vi "Stage_enable.vi"(8 "error in (no error)":errorcluster, 9 "Boolean":bool, 10 "Axes Select":u16(ring) items=["X", "Y", "Z"], 11 "reference":refnum<k7>) -> (0 "error out":errorcluster, 3 "reference out":refnum<k7>)   [LabVIEW 2020]
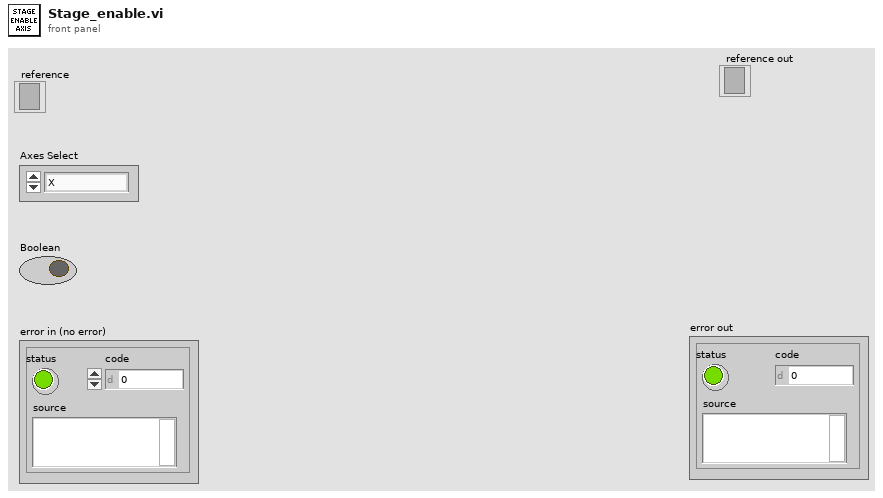
[diagram p1: front panel]
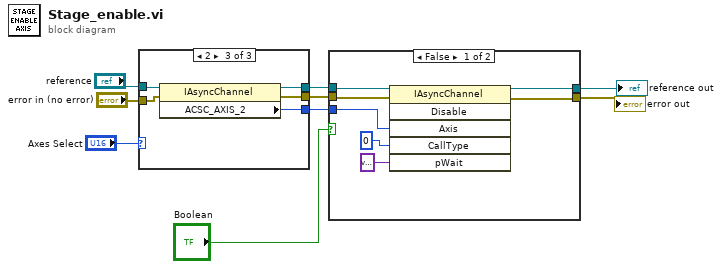
[diagram p0: block diagram]
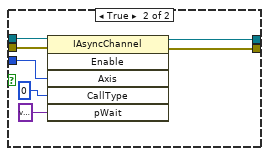
[diagram p2: hidden frame]
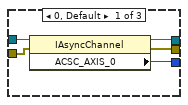
[diagram p3: hidden frame]
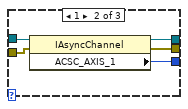
[diagram p4: hidden frame]
diagram:
  n1 = case shown="2" "Axes Select" {
    tunnel: [w14 w19 w24] -> w6
    tunnel: [w13 w18 w23] -> w5
    tunnel: [w12 w17 w22] -> w4
    tunnel: "reference" -> [w11 w16 w21]
    tunnel: "error in (no error)" -> [w10 w15 w20]
    frame 0, Default {
      n2 = property class="IAsyncChannel"(reference=w11, error in=w10) -> (reference out=w14:refnum<k7>, error out=w13:errorcluster, "ACSC_AXIS_0"=w12:i32)
    }
    frame 1 {
      n3 = property class="IAsyncChannel"(reference=w16, error in=w15) -> (reference out=w19:refnum<k7>, error out=w18:errorcluster, "ACSC_AXIS_1"=w17:i32)
    }
    frame 2 {
      n4 = property class="IAsyncChannel"(reference=w21, error in=w20) -> (reference out=w24:refnum<k7>, error out=w23:errorcluster, "ACSC_AXIS_2"=w22:i32)
    }
  }
  n5 = case shown="False" "Boolean" {
    tunnel: [w29 w36] -> w9
    tunnel: [w28 w35] -> w8
    tunnel: w6 -> [w27 w34]
    tunnel: w5 -> [w26 w33]
    tunnel: w4 -> [w25 w32]
    frame False {
      n6 = invoke class="IAsyncChannel" method="Disable"(reference=w27, error in=w26, "Axis"=w25, "CallType"=u64 0, "pWait"=variant) -> (reference out=w29:refnum<k7>, error out=w28:errorcluster)  [unwired: 1 in, 4 out]
    }
    frame True {
      n7 = invoke class="IAsyncChannel" method="Enable"(reference=w34, error in=w33, "Axis"=w32, "CallType"=u64 0, "pWait"=variant) -> (reference out=w36:refnum<k7>, error out=w35:errorcluster)  [unwired: 1 in, 4 out]
    }
  }
  "reference out" <- w9
  "error out" <- w8
